vi "AttrMapToCluster.vi"(6 "lower case Key?(F)":bool, 7 "Prototype":variant, 8 "error in (no error)":errorcluster, 11 "AttrMap":variant) -> (0 "error out":errorcluster, 3 "Cluster":variant)   [LabVIEW 2019, in "lv-apt-json-file.lvlib"]
uses:
  lv-apt-json-file.lvlib
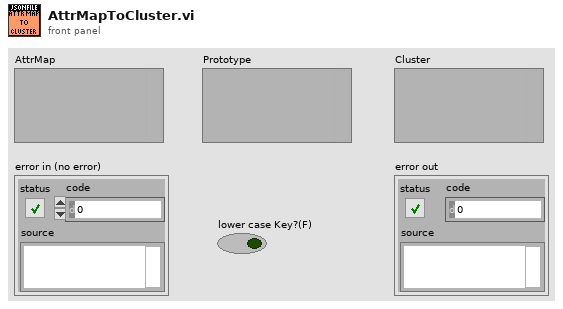
[diagram p1: front panel]
types:
  T1 = typedef "Type Descriptor Enumeration__ogtk.ctl" = enum8{"<Null>", "I8", "I16", "I32", "I64", "U8", "U16", "U32", "U64", "SGL", "DBL", "EXT", "CSG", "CDB", "CXT", "0x0F", "0x10", "0x11", "0x12", "0x13", "0x14", "Enum U8", "Enum U16", "Enum U32", "Enum U64", "SGL PQ", "DBL PQ", "EXT PQ", "CSG PQ", "CDB PQ", "CXT PQ", "0x1F", "0x20", "Boolean", "0x22", "0x23", "0x24", "0x25", "0x26", "0x27", "0x28", "0x29", "0x2A", "0x2B", "0x2C", "0x2D", "0x2E", "0x2F", "String", "0x31", "Path", "Pict", "0x34", "0x35", "0x36", "DAQ", "0x38", "0x39", "0x3A", "0x3B", "0x3C", "0x3D", "0x3E", "0x3F", "Array", "0x41", "0x42", "0x43", "0x44", "0x45", "0x46", "0x47", "0x48", "0x49", "0x4A", "0x4B", "0x4C", "0x4D", "0x4E", "0x4F", "Cluster", "0x51", "0x52", "Variant", "Waveform", "0x55", "0x56", "0x57", "0x58", "0x59", "0x5A", "0x5B", "0x5C", "0x5D", "0x5E", "0x5F", "0x60", "0x61", "0x62", "0x63", "0x64", "0x65", "0x66", "0x67", "0x68", "0x69", "0x6A", "0x6B", "0x6C", "0x6D", "0x6E", "0x6F", "Refnum"}
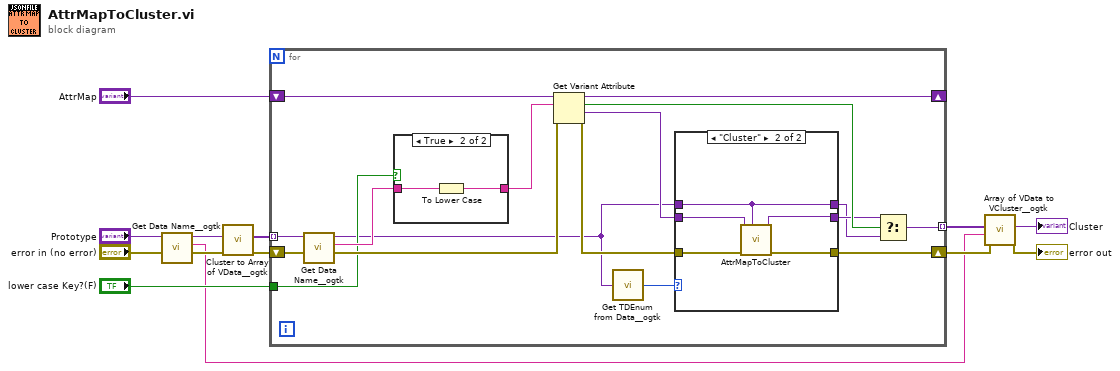
[diagram p0: block diagram]
diagram:
  n1 = call <userlib>:"Get Data Name__ogtk.vi"("error in (no error)"="error in (no error)", "Data"="Prototype") -> ("error out"=w2:errorcluster, "Data Name"=w1:string, "Data dup"=w4:variant)  [unwired: 7 in]
  n2 = call <userlib>:"Cluster to Array of VData__ogtk.vi"("error in (no error)"=w2, "Cluster"=w4) -> ("error out"=w13:errorcluster, "Array of VData"=w12:variant[])  [unwired: 8 in]
  n3 = for {
    tunnel: w12 -> [w27] mode=indexing
    shift-right: [w29] -> _
    shift-left: "AttrMap" -> [w30]
    shift-right: [w16] -> w8
    shift-left: w13 -> [w26]
    tunnel: "lower case Key?(F)" -> [w23]
    tunnel: [w21] -> w9 mode=indexing
    n4 = call <userlib>:"Get Data Name__ogtk.vi"("error in (no error)"=w26, "Data"=w27) -> ("error out"=w25:errorcluster, "Data Name"=w28:string, "Data dup"=w15:variant)  [unwired: 7 in]
    n5 = case shown="True" w23 {
      tunnel: w28 -> [w39 w41]
      tunnel: [w39 w40] -> w24
      frame False {
      }
      frame True {
        n6 = To Lower Case(string=w41) -> (all lower case string=w40:string)
      }
    }
    n7 = Get Variant Attribute(Variant=w30, name=w24, error in=w25) -> (duplicate Variant=w29:variant, found=w22:bool, value=w19:variant, error out=w17:errorcluster)  [unwired: 1 in]
    n8 = call <userlib>:"Get TDEnum from Data__ogtk.vi"("Data"=w15) -> ("Type Descriptor Enumeration"=w20:T1)  [unwired: 4 in]
    n9 = case shown="\"Cluster\"" w20 {
      tunnel: w19 -> [w33 w38]
      tunnel: [w33 w37] -> w18
      tunnel: w17 -> [w31 w36]
      tunnel: [w31 w35] -> w16
      tunnel: w15 -> [w32 w34]
      tunnel: [w32 w34] -> w14
      frame Default {
      }
      frame "Cluster" {
        n10 = call "AttrMapToCluster.vi"("Prototype"=w34, "error in (no error)"=w36, "AttrMap"=w38) -> ("error out"=w35:errorcluster, "Cluster"=w37:variant)  [unwired: 7 in]
      }
    }
    n11 = Select(t=w18, s=w22, f=w14) -> (s? t:f=w21:variant)
  }
  n12 = call <userlib>:"Array of VData to VCluster__ogtk.vi"("error in (no error)"=w8, "Cluster Name"=w1, "Array"=w9) -> ("error out"=→"error out":errorcluster, "VCluster"=→"Cluster":variant)  [unwired: 7 in]
